vi "Spawn Write Process.vi"(8 "error in (no error)":errorcluster, 11 "DbMeasurement in":refnum<class "DbMeasurement.lvclass">) -> (0 "error out":errorcluster, 3 "DbMeasurement out":refnum<class "DbMeasurement.lvclass">)   [LabVIEW 2013, in "DbMeasurement.lvclass"]
doc: "This method spawns the write data method as a separate process. The write data method then runs as long as the data queue exists."
uses:
  DbMeasurement.lvclass
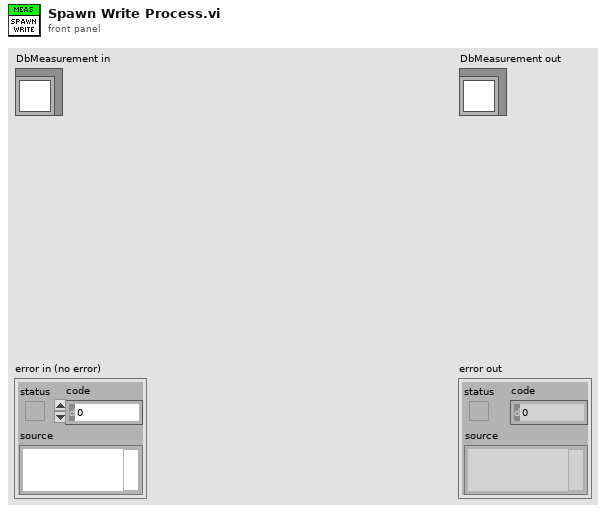
[diagram p1: front panel]
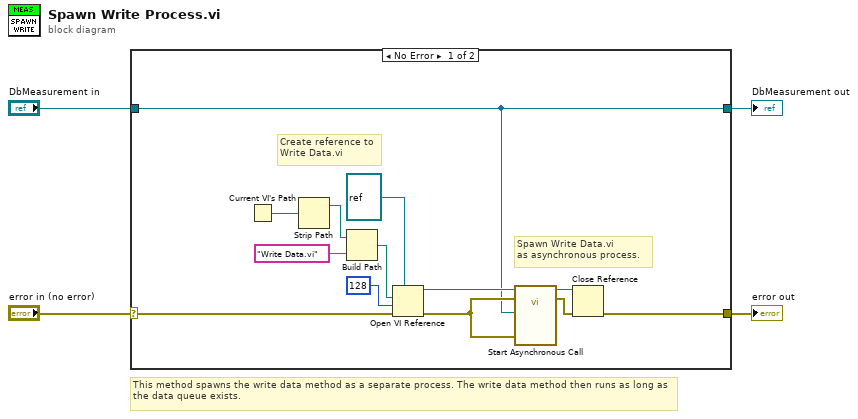
[diagram p0: block diagram]
diagram:
  # "This method spawns the write data method as a separate process. The write data method then runs as long as the data queue exists."
  n1 = case shown="No Error" "error in (no error)" {
    selector: "error in (no error)" -> [w7 w19]
    tunnel: [w6 w19] -> w3
    tunnel: [w5 w18] -> w1
    tunnel: "DbMeasurement in" -> [w5 w18]
    frame No Error {
      # "Spawn Write Data.vi\nas asynchronous process."
      # "Create reference to\nWrite Data.vi"
      n2 = Current VI's Path() -> (path=w17:path)
      n3 = Strip Path(path=w17) -> (stripped path=w16:path)  [unwired: 1 out]
      n4 = Build Path(base path=w16, name or relative path="Write Data.vi") -> (appended path=w14:path)
      n5 = Open VI Reference(type specifier VI Refnum (for type only)=refnum<vi> refnum, vi path=w14, options=128, error in (no error)=w7) -> (vi reference=w9:refnum<vi>, error out=w8:errorcluster)  [unwired: 2 in]
      n6 = call-by-ref "Start Asynchronous Call"(reference=w9, error in=w8, 8:"error in (no error)"=w8, "DbMeasurement in 2"=w5) -> (reference out=w12:refnum<vi>, error out=w11:errorcluster)  [unwired: 8 in, 2 out]
      n7 = Close Reference(reference=w12, error in (no error)=w11) -> (error out=w6:errorcluster)
    }
    frame Error {
    }
  }
  "error out" <- w3
  "DbMeasurement out" <- w1
